vi "Release Logs Queue.vi"(8 "Error In":errorcluster, 11 "EventLog in":refnum<class "EventLog.lvclass">) -> (0 "Error Out":errorcluster, 3 "EventLog out":refnum<class "EventLog.lvclass">)   [LabVIEW 2019, in "EventLog.lvlib" / "EventLog.lvclass"]
uses:
  EventLog.lvclass
  EventLog.lvclass/EventLog.ctl
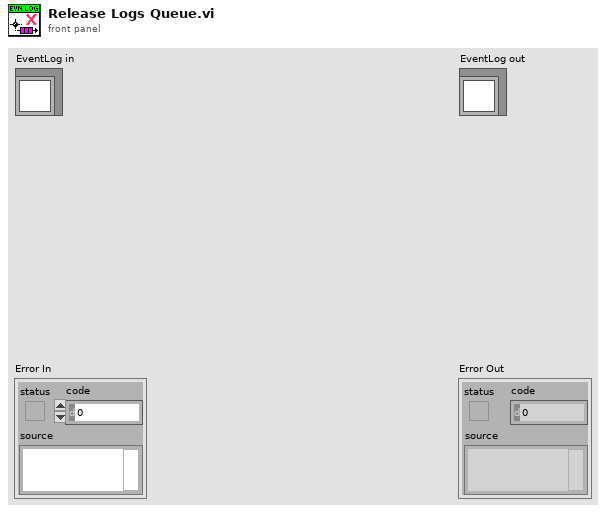
[diagram p1: front panel]
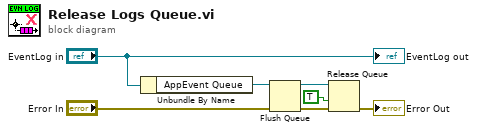
[diagram p0: block diagram]
diagram:
  n1 = Unbundle By Name("EventLog in") -> ("AppEvent Queue"=w4:refnum<queue>)
  n2 = Flush Queue(queue=w4, error in (no error)="Error In") -> (queue out=w3:refnum<queue>, error out=w2:errorcluster)  [unwired: 1 out]
  n3 = Release Queue(queue=w3, force destroy? (F)=TRUE, error in (no error)=w2) -> (error out=→"Error Out":errorcluster)  [unwired: 2 out]
  "EventLog out" <- "EventLog in"
